vi "PmacCommGetBuffer.vi"(0 "Device Number i32 (0)":i32 min=0) -> (1 "Response Available Bool (F)":bool, 2 "Response String (\"\")":string)   [LabVIEW 2020]
doc: "Check if PMAC has data available. When Response Available is TRUE Response String contains all available data. When Response Available is FALSE Response String is the empty string. Responses are not parsed for PMAC ERR codes.\n\nThis VI is used by PmacCommGetResponse and PmacCommGetStr to retrieve very large response buffers. These two VIs are limited by PComm32 to responses of 256 characters whereas this VI is not. You will not generally use this VI."
uses:
  Builds/5-8-13/data/PComm32W.dll
panel:
  in  "NumChars":u32
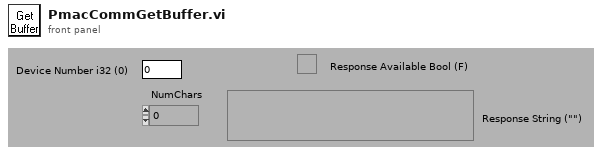
[diagram p1: front panel]
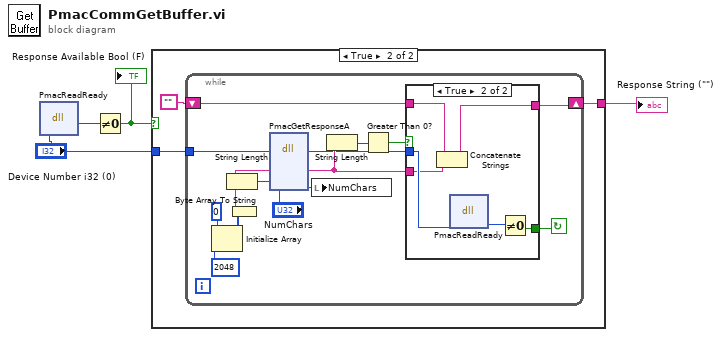
[diagram p0: block diagram]
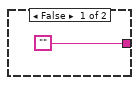
[diagram p2: hidden frame]
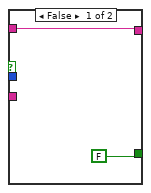
[diagram p3: hidden frame]
diagram:
  n1 = dll-call lib="C:/NUWAR_Master/Builds/5-8-13/data/PComm32W.dll" fn="PmacReadReady" label="DeviceReadReady"("DeviceNumber"="Device Number i32 (0)") -> (w4:u32)  [unwired: 4 in, 2 out]
  n2 = Not Equal To 0?(x=w4) -> (x != 0?=w3:bool)
  "Response Available Bool (F)" <- w3
  n3 = case shown="True" w3 {
    tunnel: "Device Number i32 (0)" -> [_ w8]
    tunnel: ["" w6] -> w1
    frame False {
    }
    frame True {
      n4 = while {
        shift-left: "" -> [w21]
        shift-right: [w20] -> w6
        tunnel: w8 -> [w9]
        stop <- w15 continue-if-true
        n5 = Initialize Array(u8 0, 2048) -> (w16:u8[])
        n6 = Byte Array To String(unsigned byte array=w16) -> (string=w14:string)
        n7 = String Length(string=w14) -> (length=w13:i32)
        n8 = dll-call lib="C:/NUWAR_Master/Builds/5-8-13/data/PComm32W.dll" fn="PmacGetResponseA" ("PmacBUSGetBuffer")("DeviceNumber"=w9, "Response"=w14, "MaxChar"=w13, "CharsRead"="NumChars") -> ("Response"=w10:string, "CharsRead"=w11:u32)  [unwired: 5 in, 3 out]
        n9 = local write "NumChars"(w11) -> ()
        n10 = String Length(string=w10) -> (length=w22:i32)
        n11 = Greater Than 0?(x=w22) -> (x > 0?=w19:bool)
        n12 = case shown="True" w19 {
          tunnel: w21 -> [w24 w30]
          tunnel: [w24 w29] -> w20
          tunnel: [FALSE w27] -> w15
          tunnel: w9 -> [_ w26]
          tunnel: w10 -> [_ w25]
          frame False {
          }
          frame True {
            n13 = Concatenate Strings(w30, w25) -> (w29:string)
            n14 = dll-call lib="C:/NUWAR_Master/Builds/5-8-13/data/PComm32W.dll" fn="PmacReadReady" label="DeviceReadReady"("DeviceNumber"=w26) -> ("DeviceNumber"=w28:i32)  [unwired: 3 in, 3 out]
            n15 = Not Equal To 0?(x=w28) -> (x != 0?=w27:bool)
          }
        }
      }
    }
  }
  "Response String (\"\")" <- w1
